vi "指令-修改报警限值-网络版-1001版.vi"(11 "限值":dbl format="%#_13g") -> (3 "指令输出":string)   [LabVIEW 2017]
uses:
  <vilib>/regexp/Match Regular Expression.xnode
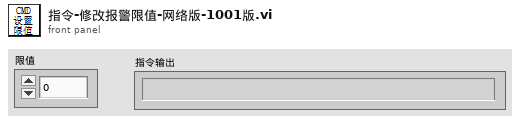
[diagram p1: front panel]
types:
  T1 = typedef "簇-输入.ctl" = cluster{"配置文件动作":T2, "数据输入":variant}
  T2 = typedef "枚举-配置文件动作.ctl" = enum16{"初始化加载配置", "读取配置", "写入-屏幕键盘", "写入-静音延迟", "写入-主要探头类型", "写入-串口配置", "写入-累积定时", "写入-导出定时", "保存配置到文件"}
  T3 = typedef "簇-配置文件内容.ctl" = cluster{"调试模式？":bool, "屏幕键盘？":bool, "软件版本":string, "静音延迟 s":u16, "主要探头类型":T4, "串口配置":cluster{"COM口":refnum<visa-resource-name>, "波特率":enum16{"9600", "19200"}, "读写超时ms":i16, "丢包判定次数":i16}, "定时配置-累积分段":T5, "定时配置-自动导出":cluster{"定时配置-自动导出":T5, "分别导出?":bool}}
  T4 = typedef "枚举-主要探头类型.ctl" = enum16{"网络探头", "串口探头"}
  T5 = typedef "簇-定时配置.ctl" = cluster{"定时模式":enum16{"绝对时间", "相对时间"}, "单位":enum16{"年", "月", "日", "时", "分"}, "间隔":u8, "目标时刻":timestamp}
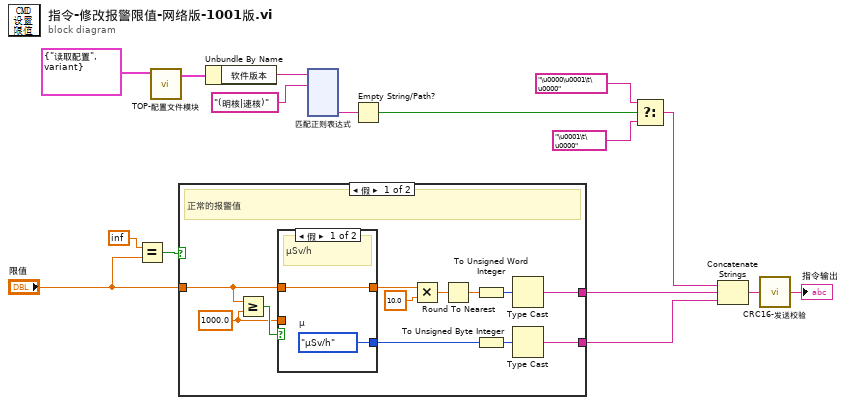
[diagram p0: block diagram]
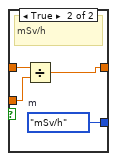
[diagram p2: hidden frame]
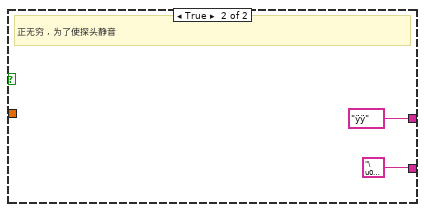
[diagram p3: hidden frame]
diagram:
  n1 = Equal?(x=inf, y="限值") -> (x = y?=w10:bool)
  n2 = call "TOP-配置文件模块.vi"("输入"=T1 {"配置文件动作"=enum."读取配置", "数据输入"=variant}) -> ("配置文件"=w4:T3)  [unwired: 9 in, 1 out]
  n3 = case shown="假" w10 {
    tunnel: [w19 "\u0001"] -> w15
    tunnel: [w18 "ÿÿ"] -> w13
    tunnel: "限值" -> [w17 _]
    frame False {
      w27 = 1000.0 ("y")
      # "正常的报警值"
      n4 = Greater Or Equal?(x=w17, y=w27) -> (x >= y?=w28:bool)
      n5 = case shown="假" w28 {
        tunnel: w17 -> [w29 w33]
        tunnel: [w30 w34] -> w21
        tunnel: w27 -> [_ w32]
        tunnel: [w29 w31] -> w26
        frame False {
          w30 = enum8{"μSv/h", "mSv/h"}."μSv/h"  # μ
          # "μSv/h"
        }
        frame True {
          w34 = enum8{"μSv/h", "mSv/h"}."mSv/h"  # m
          # "mSv/h"
          n6 = Divide(x=w33, y=w32) -> (x/y=w31:dbl)
        }
      }
      n7 = Multiply(x=w26, y=10.0) -> (x*y=w23:dbl)
      n8 = Round To Nearest(number=w23) -> (nearest integer value=w22:dbl)
      n9 = To Unsigned Word Integer(number=w22) -> (unsigned 16bit integer=w24:u16)
      n10 = To Unsigned Byte Integer(number=w21) -> (unsigned 8bit integer=w20:u8)
      n11 = Type Cast(x=w24) -> (*(type *) &x=w18:string)  [unwired: 1 in]
      n12 = Type Cast(x=w20) -> (*(type *) &x=w19:string)  [unwired: 1 in]
    }
    frame True {
      # "正无穷 , 为了使探头静音"
    }
  }
  n13 = Unbundle By Name(w4) -> ("软件版本"=w3:string)
  n14 = xnode "匹配正则表达式"("输入字符串"=w3, "正则表达式"="(明核|速核)") -> ("子匹配 1"=w2:string)  [unwired: 4 in, 5 out]
  n15 = Empty String/Path?(string/path=w2) -> (empty?=w1:bool)
  n16 = Select(t="\u0000\u0001\t\u0000", s=w1, f="\u0001\t\u0000") -> (s? t:f=w7:string)
  n17 = Concatenate Strings(w7, w13, w15) -> (w16:string)
  n18 = call "CRC16-发送校验.vi"("净数据"=w16) -> ("完整输出"=→"指令输出":string)
